vi "SW_Generate_Segmented_Plot_v3.vi"(5 "Regions to mark selected":u16[](array[numeric]), 7 "Regions to mark set":u16[](array[numeric]), 9 "Show magnets":bool=TRUE, 10 "Input cluster of parameters":T2={"Amount of border segments"=8, "Border segments starting angle"=0, "Amount of midfield segments"=4, "Midfield segments starting angle"=0, "Midfield segments outer radius, mm"=60, "Amount of central segments"=1, "Center segment outer radius, mm"=30, "Diameter of the cage, mm"=180, "R-gap between segments, mm"=10} {"Diameter of the cage, mm" scale=20.0..250.0}, 11 "Draw Area Size":cluster{"Width":dbl, "Height":dbl}={"Width"=480.0, "Height"=480.0}) -> (0 "Array of the pixel to color correspondences":u32[][](array[numeric]), 1 "Array of the segment to color correspondences":u32[][](array[numeric]), 2 "No zones image":picture, 3 "Zones layout output":picture)   [LabVIEW 2016]
panel:
  out "Colors cluster":T1={"Colors array for outer segments"=[14102567, 16625249, 14742520, 7646673, 16018755, 16703632, 11262441, 4552116], "Colors array for midfield segments"=[8073876, 10935200, 34871, 12756431], "Color for central segment"=16777113, "Fill color for no segments image"=6316128}
  out "Zones display background":picture
  in  "Scale factor for outer display radius display":dbl=0.95 format="%#_13g"
  in  "Fill color for no segments image":u32(colorbox)=6316128
  out "Error Out":errorcluster
  in  "Error In":errorcluster
  in  "Color for central segment":u32=16777113
  in  "Colors array for midfield segments":u32[](array[numeric])=[8073876, 10935200, 34871, 12756431]
  in  "Colors array for outer segments":u32[](array[numeric])=[14102567, 16625249, 14742520, 7646673, 16018755, 16703632, 11262441, 4552116]
  in  "Background color":u32(colorbox)=13816530
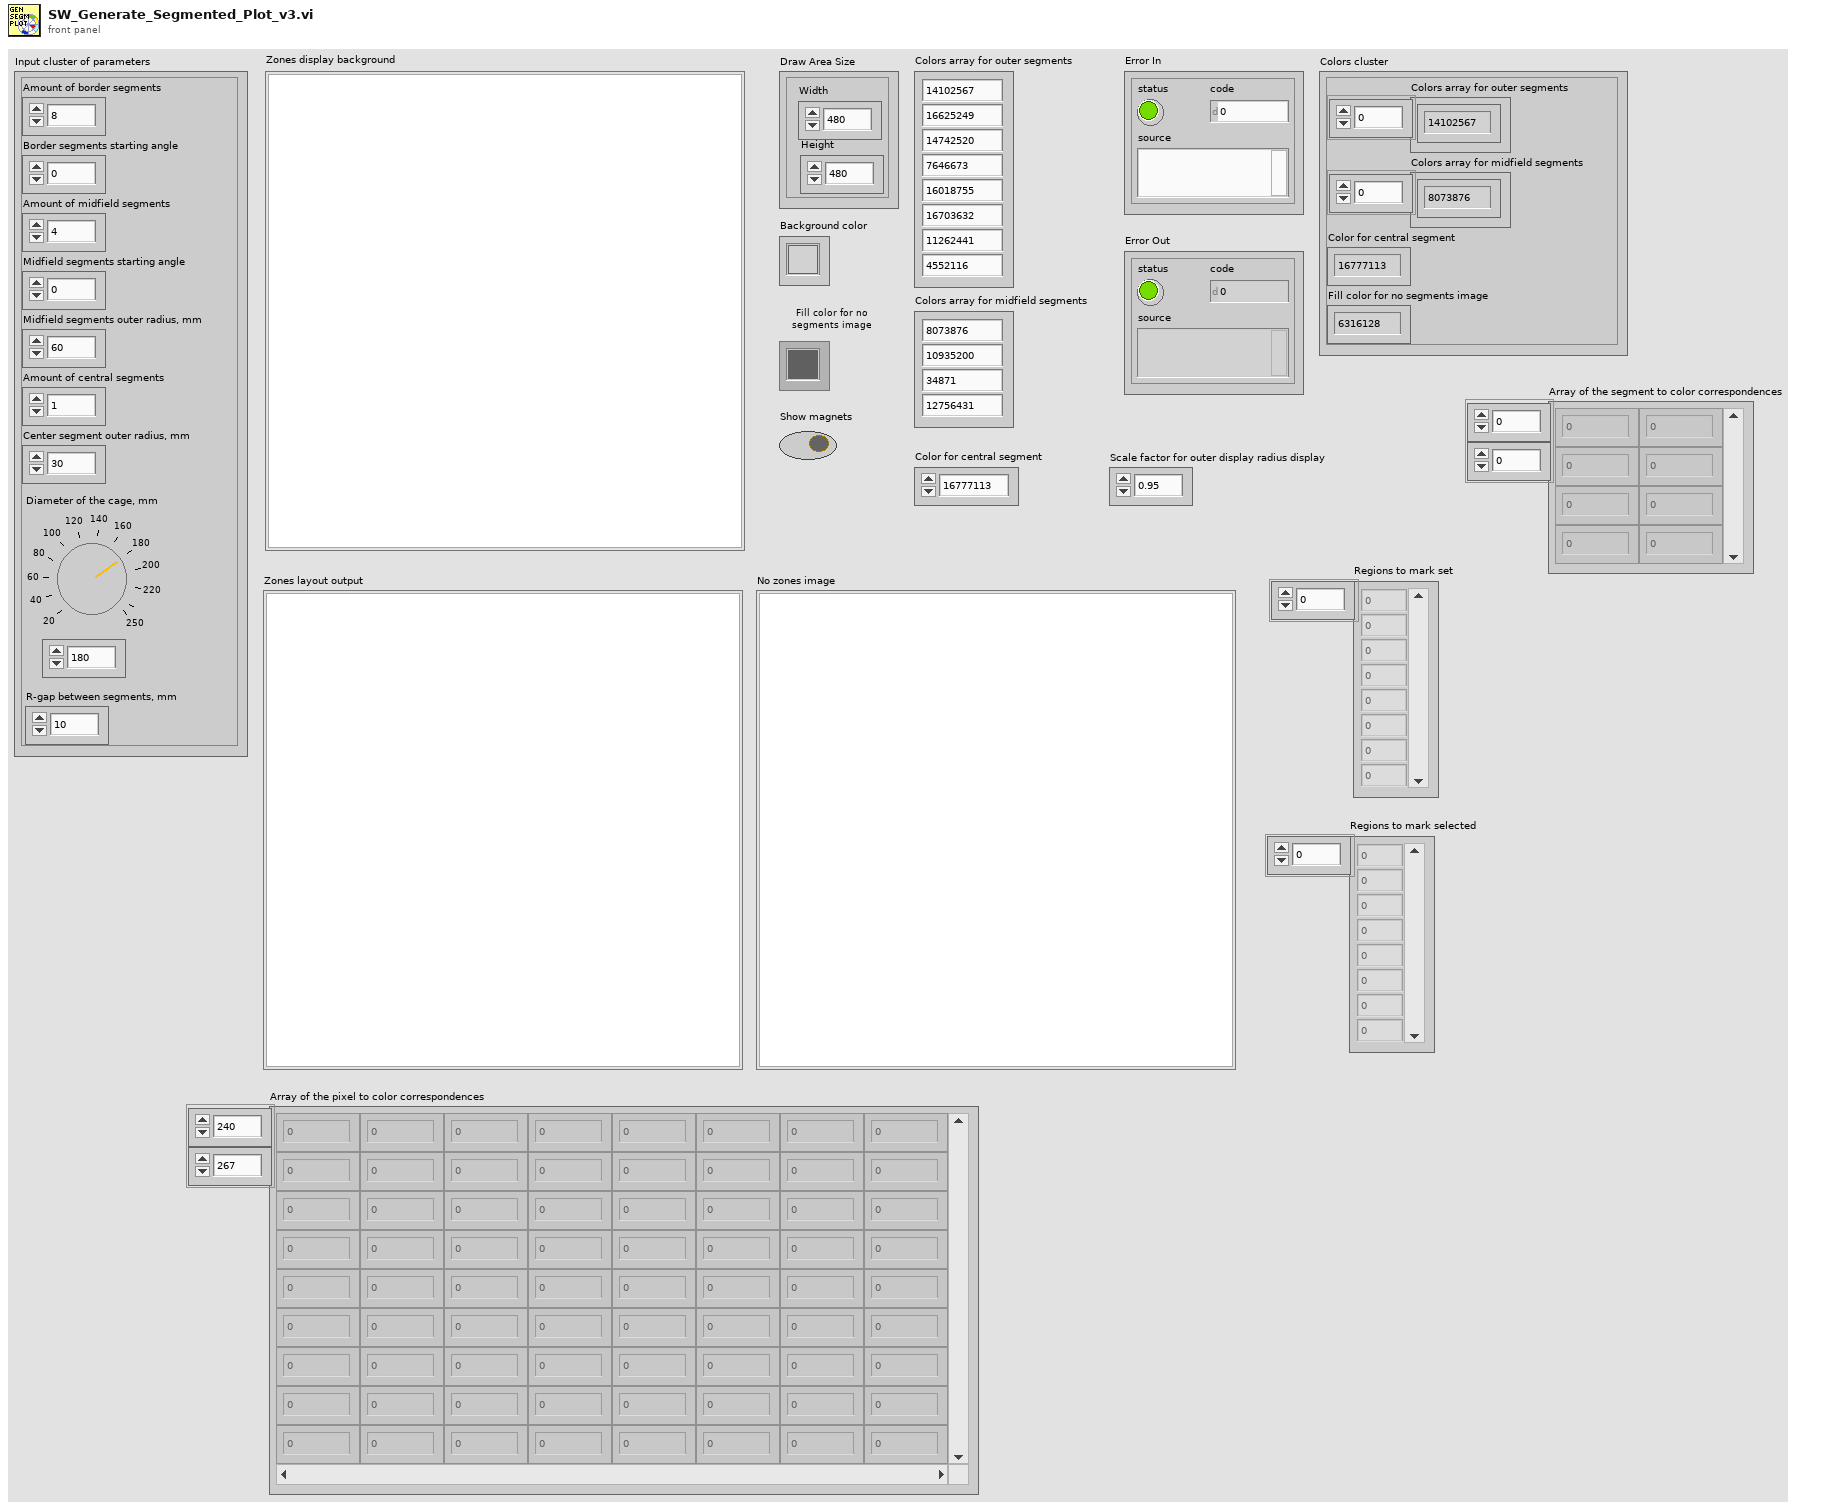
[diagram p1: front panel]
types:
  T1 = cluster{"Colors array for outer segments":u32[], "Colors array for midfield segments":u32[], "Color for central segment":u32, "Fill color for no segments image":u32}
  T2 = cluster{"Amount of border segments":u8, "Border segments starting angle":i16, "Amount of midfield segments":u8, "Midfield segments starting angle":i16, "Midfield segments outer radius, mm":u16, "Amount of central segments":u8, "Center segment outer radius, mm":u16, "Diameter of the cage, mm":u16, "R-gap between segments, mm":u8}
  T3 = cluster{"Fonts scale factor":dbl, "Pixels per mm":dbl, "Radius of displayed outer segments, pix":dbl, "Radius of displayed midfield segments, pix":dbl, "Radius of displayed central segment, pix":dbl}
  T4 = cluster{"Bounding rectangle for outer segments, pix":cluster{"TL W, pix":dbl, "TL H, pix":dbl, "RB W, pix":dbl, "RB H, pix":dbl}, "Bounding rectangle of the midfield segments, pix":cluster{"TL W, pix":dbl, "TL H, pix":dbl, "RB W, pix":dbl, "RB H, pix":dbl}, "Coordinates of the center of the image, pix":cluster{"W, pix":dbl, "H, pix":dbl}}
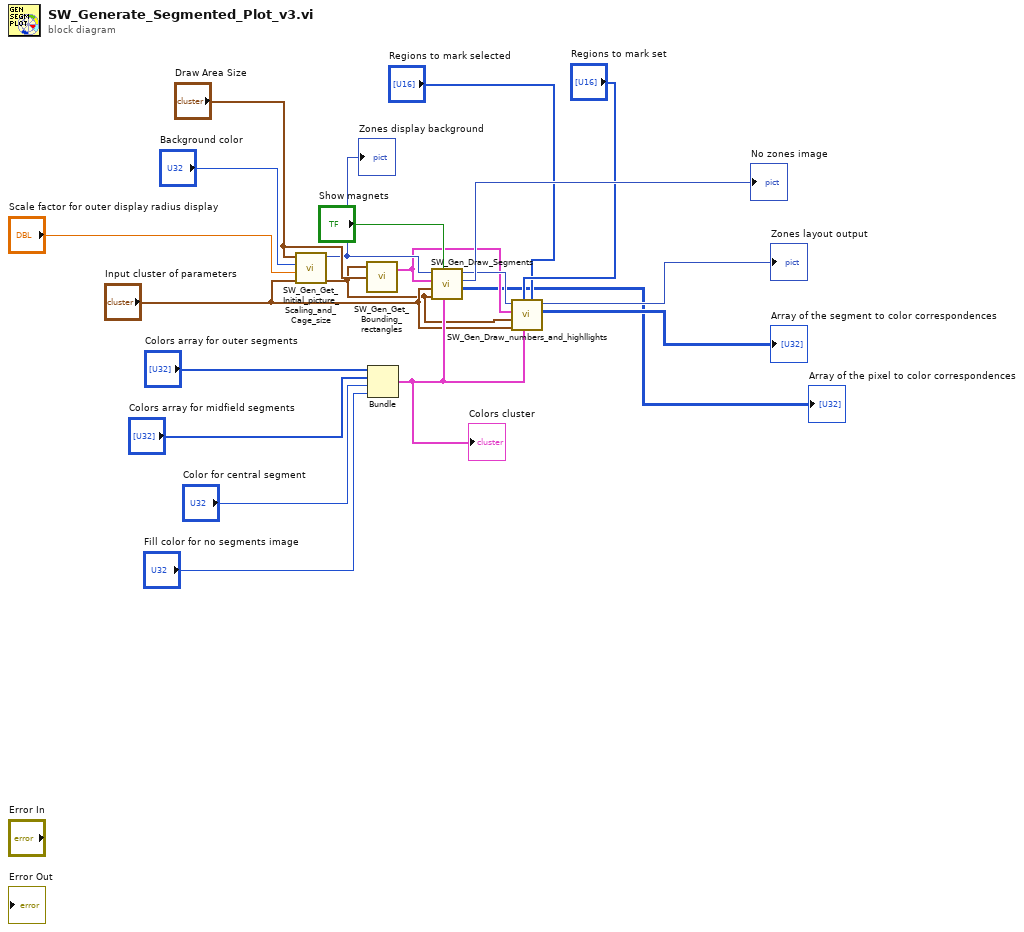
[diagram p0: block diagram]
diagram:
  n1 = call "SW_Gen_Get_Initial_picture_Scaling_and_Cage_size.vi"("Input cluster of parameters"="Input cluster of parameters", "Scale factor for outer display radius display"="Scale factor for outer display radius display", "Background color"="Background color", "Draw Area Size"="Draw Area Size") -> ("Cluster of image geometrical and scaling parameters"=w6:T3, "Zones display background"=w17:picture)  [unwired: 6 in]
  "Zones display background" <- w17
  n2 = call "SW_Gen_Get_Bounding_rectangles.vi"("Draw Area Size"="Draw Area Size", "Cluster of image geometrical and scaling parameters"=w6) -> ("Bounding rectangles"=w5:T4)  [unwired: 2 in]
  n3 = Bundle("Colors array for outer segments"="Colors array for outer segments", "Colors array for midfield segments"="Colors array for midfield segments", "Color for central segment"="Color for central segment", "Fill color for no segments image"="Fill color for no segments image") -> (w8:T1)  [unwired: 1 in]
  "Colors cluster" <- w8
  n4 = call "SW_Gen_Draw_Segments.vi"("Colors cluster"=w8, "Show magnets"="Show magnets", "Cluster of image geometrical and scaling parameters"=w6, "Input cluster of parameters"="Input cluster of parameters", "Bounding rectangles"=w5, "Zones display background in"=w17) -> ("Array of the pixel to color correspondences"=→"Array of the pixel to color correspondences":u32[][], "No zones image"=→"No zones image":picture, "Zones in the cage layout"=w10:picture)  [unwired: 3 in]
  n5 = call "SW_Gen_Draw_numbers_and_highllights.vi"("Regions to mark selected"="Regions to mark selected", "Colors cluster"=w8, "Regions to mark set"="Regions to mark set", "Input cluster of parameters"="Input cluster of parameters", "Cluster of image geometrical and scaling parameters"=w6, "Bounding rectangles"=w5, "Zones layout input"=w10) -> ("Array of the segment to color correspondences"=→"Array of the segment to color correspondences":u32[][], "Zones layout output"=→"Zones layout output":picture)  [unwired: 3 in]
